vi "InitialiseProbeplan.vi"() -> ()   [LabVIEW 2018]
doc: "General utility to initialise, generate, test and execute probe plans."
uses:
  general_VIs/globals/QC_MeasurementSetup.vi
  ProbePlanParams.vi
  InstrControl/ProbeStationControl/ProbeStationControl.lvclass
panel:
  in  "Use index as X coord":bool=TRUE
  in  "Continue":bool
  in  "New Sensor":bool
  in  "Single Needle":bool=TRUE
  out "Chuck Up/Down check":bool
  in  "Probe Card Channels":i32=1
  in  "Strip No.":u16(ring)
  out "Probeplan:":string="- Click 'New' to load new Probeplan\n- Use controls to check alignment"
  in  "Region":u16(ring)
  in  "Chuck":bool caption="Chuck\nDOWN"
  in  "New Button":bool
  in  "Jump Button":bool
  # "Probeplan"
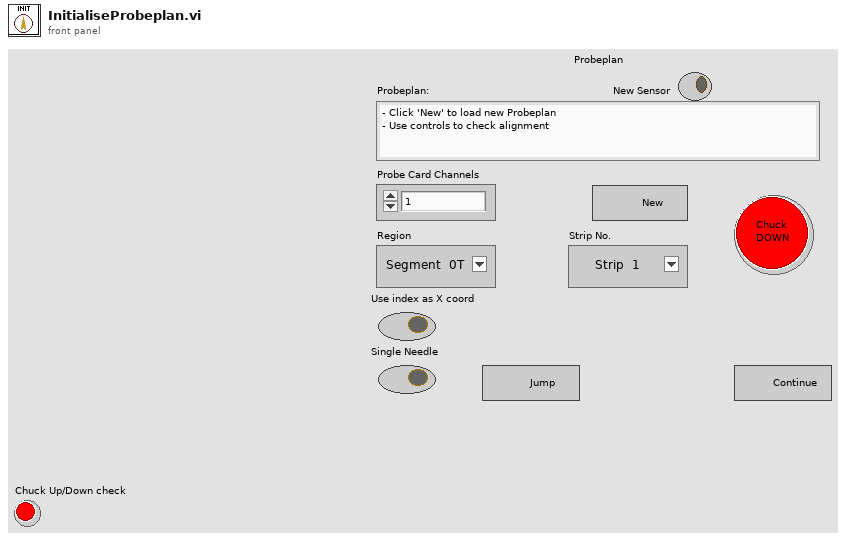
[diagram p1: front panel]
types:
  T1 = cluster{"Bias Supply":refnum<class "SupplyControl.lvclass">, "SMU":refnum<class "SupplyControl.lvclass">, "LCR":refnum<class "LCRControl.lvclass">, "Probe Card Channels":i32, "Bias Voltage [V]":dbl, "First strip":i32, "Last strip":i32, "Base Voltage [V]":dbl, "Base Ramp Step [V]":dbl, "Base Ramp Interval [ms]":u32, "High Voltage [V]":dbl, "High Ramp Step [V]":dbl, "High Ramp Interval [ms]":u32, "Single Needle":bool, "Temperature Readout":enum16{"Read Arduino", "Enter manually"}, "Arduino":refnum<class "ArduinoControl.lvclass">, "Fraction of good strips [%]":dbl, "ProbeStation":refnum<class "ProbeStationControl.lvclass">, "AC frequency [Hz]":i32, "Switching":refnum<class "Switching.lvclass">, "Matrix used?":bool, "Matrix X Channels":cluster{"Bias Supply / SMU LO":i32, "Bias Supply / SMU HI":i32, "CV Box LO":i32, "CV Box HI":i32, "CV Box LO IN":i32, "CV Box HI IN":i32, "Volt meter LO":i32, "Volt meter HI":i32, "Mux1 C1":i32, "Mux1 C2":i32, "Mux2 C1":i32, "Mux2 C2":i32}, "Pinholes Y/N":bool, "Capacitance Y/N":bool, "Resistance Y/N":bool}
  T2 = cluster{"Strip Number OUT":i32, "X0":i32, "Y0":i32, "X1":i32, "Y1":i32, "Xref":dbl, "Yref":dbl, "ProbePlan type":u32, "Inner pads offset":ext, "Outer pads offset":ext, "l_inner":ext, "l_outer":ext, "strip numbering":u16, "Device Orientation":ext, "Stagger offset":i32, "Yoffset":dbl, "Strip pitch":dbl, "Fiducail separation":dbl, "Radius":ext, "Relative strip angles":dbl, "Probeplan description":string, "ProbePlan array":cluster{"Region":string, "ProbePoints":cluster{"X":dbl, "Y":dbl, "Label":string, "CardViable?":bool}[]}[], "Test ProbePoints":cluster{"Regions Enabled":bool[], "From index":u32[], "To index":u32[]}}
  T3 = cluster{"Region":string, "ProbePoints":cluster{"X":dbl, "Y":dbl, "Label":string, "CardViable?":bool}[]}[]
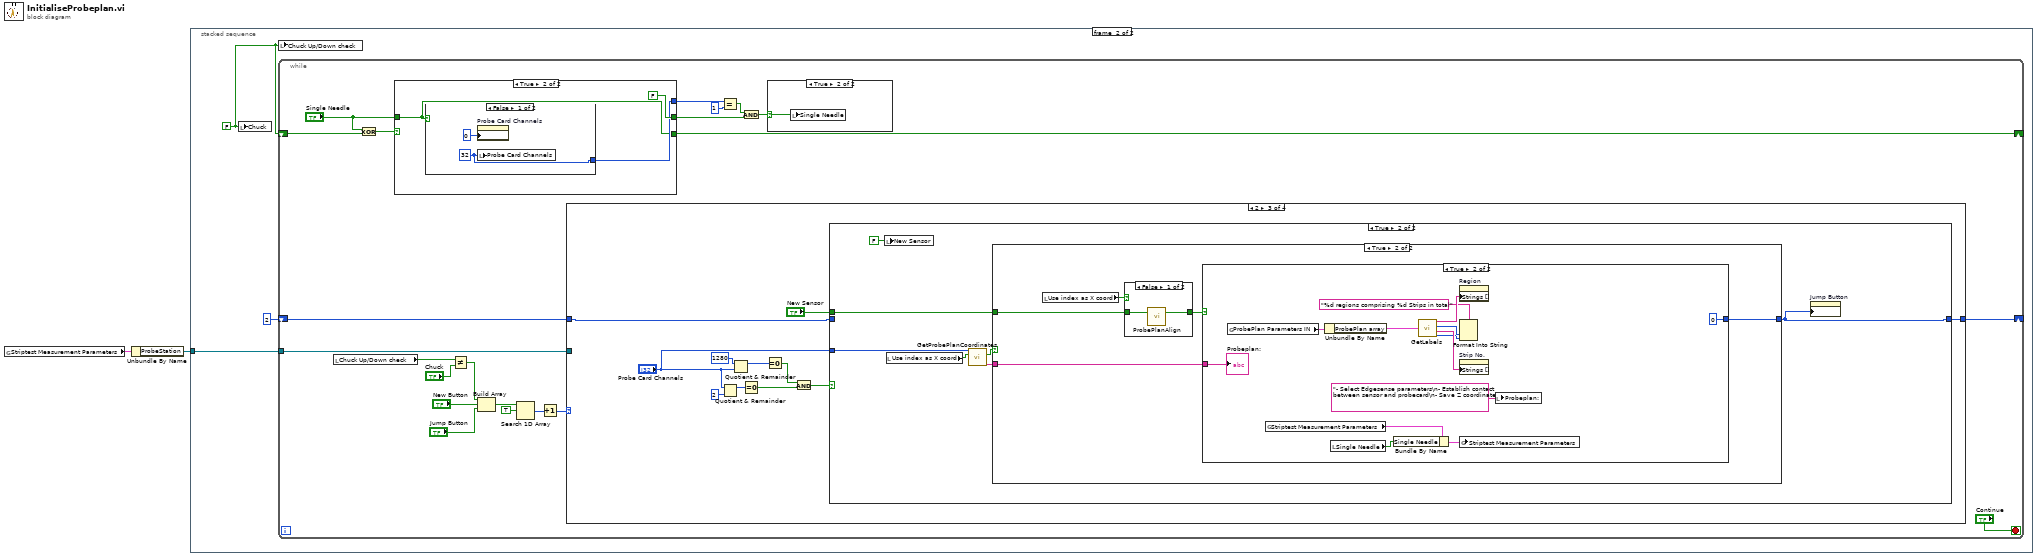
[diagram p0: block diagram]
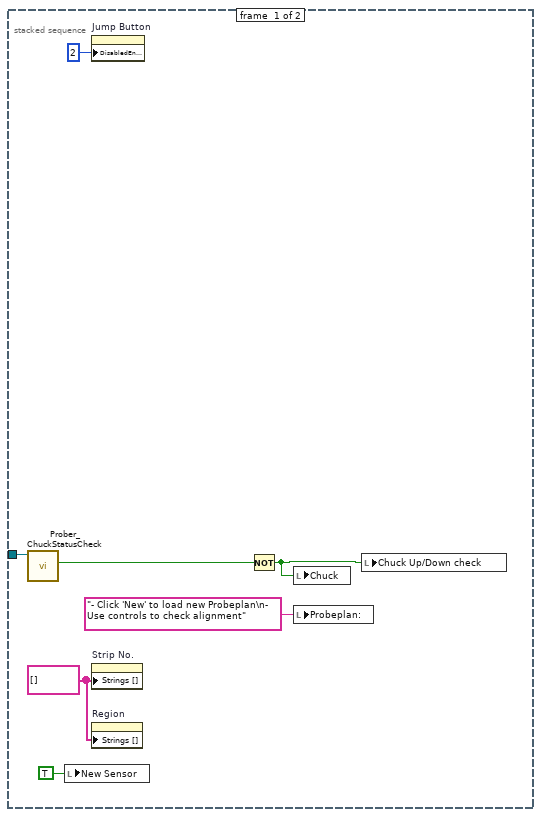
[diagram p2: hidden frame]
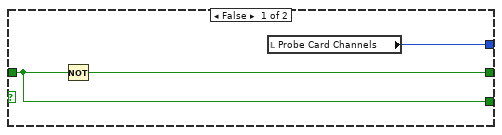
[diagram p4: hidden frame]
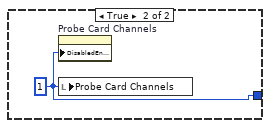
[diagram p5: hidden frame]
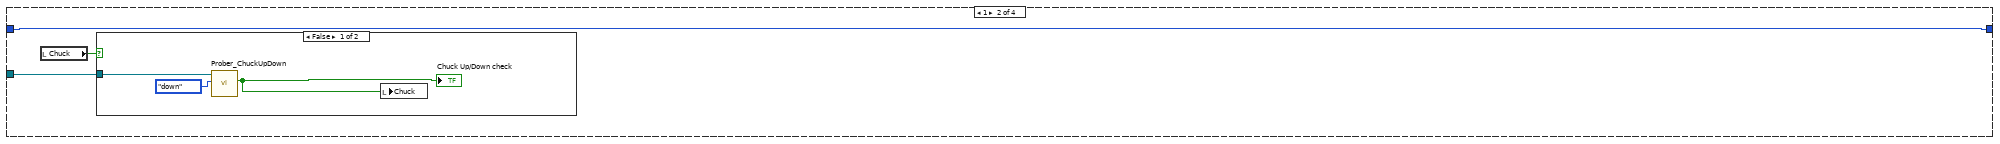
[diagram p7: hidden frame]
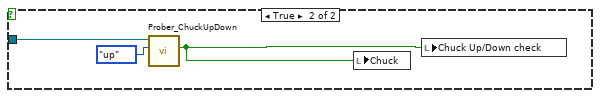
[diagram p8: hidden frame]
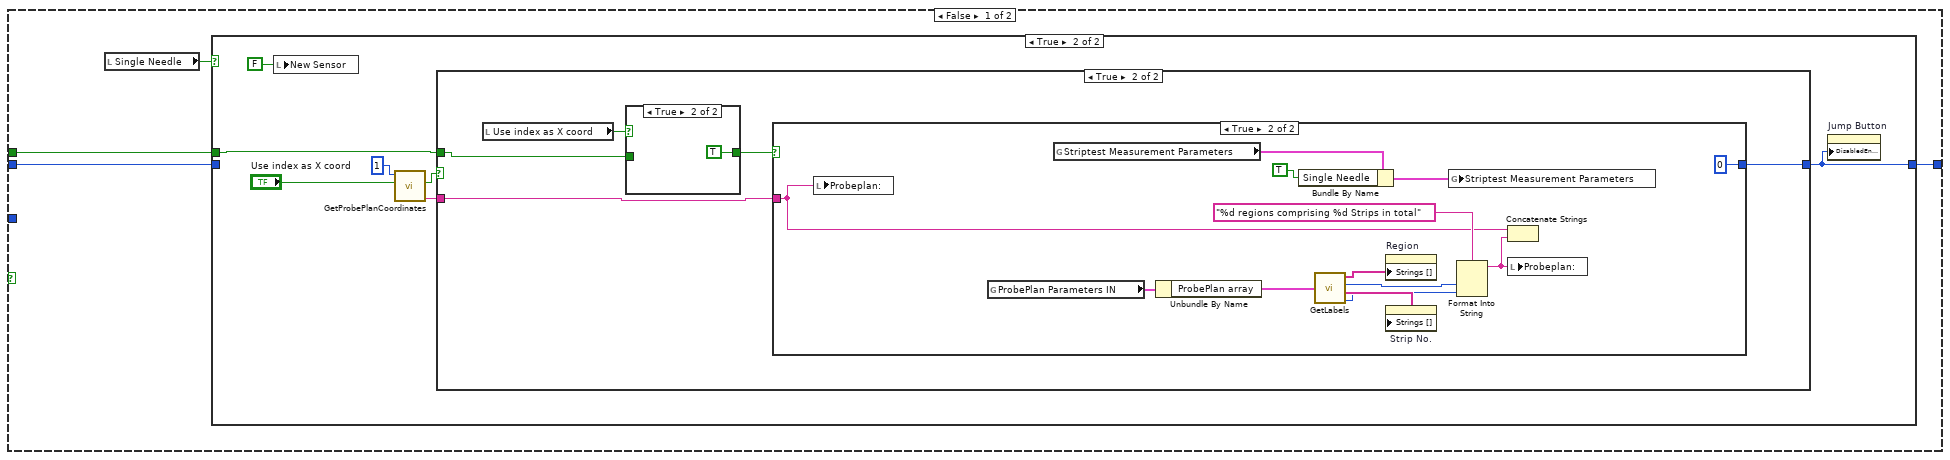
[diagram p9: hidden frame]
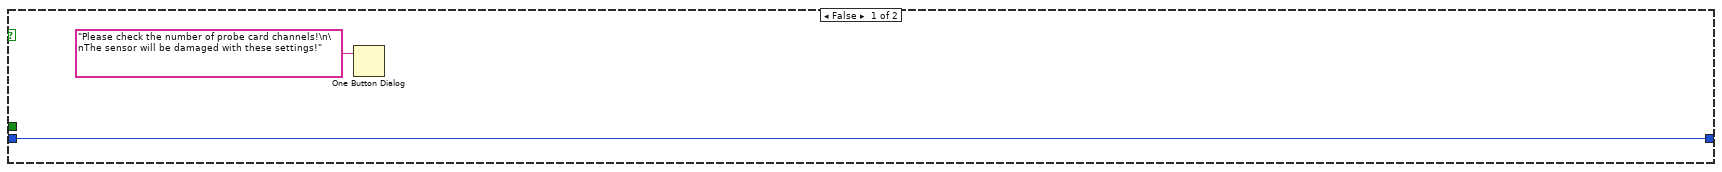
[diagram p10: hidden frame]
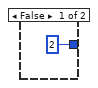
[diagram p11: hidden frame]
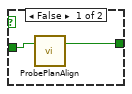
[diagram p12: hidden frame]
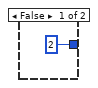
[diagram p13: hidden frame]
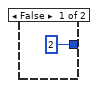
[diagram p14: hidden frame]
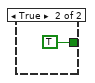
[diagram p15: hidden frame]
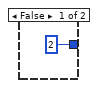
[diagram p16: hidden frame]
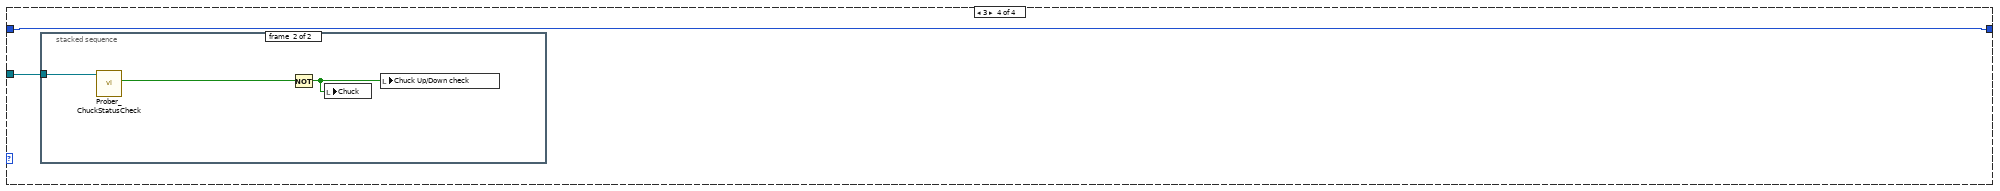
[diagram p17: hidden frame]
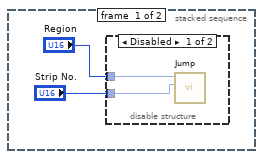
[diagram p18: hidden frame]
diagram:
  n1 = global read "QC_MeasurementSetup.vi" "Striptest Measurement Parameters"() -> (w2:T1)
  n2 = Unbundle By Name(w2) -> ("ProbeStation"=w1:refnum<class "ProbeStationControl.lvclass">)
  n3 = stacked-sequence {
    tunnel: w1 -> [w3 w10]
    frame #0 {
      w7 = string[] []
      n4 = call-dynamic "Prober_ChuckStatusCheck.vi"("ProbeStationControl in"=w3) -> ("Chuck at CONTACT?"=w5:bool)  [unwired: 8 in, 2 out]
      n5 = local write "New Sensor"(TRUE) -> ()
      n6 = property on="Jump Button" class="Bool"("DisabledEnum"=2) -> ()  [unwired: 2 in, 2 out]
      n7 = property on="Strip No." class="Ring (strict)"("Strings []"=w7) -> ()  [unwired: 2 in, 2 out]
      n8 = property on="Region" class="Ring (strict)"("Strings []"=w7) -> ()  [unwired: 2 in, 2 out]
      n9 = Not(x=w5) -> (.not. x?=w4:bool)
      n10 = local write "Chuck"(w4) -> ()
      n11 = local write "Probeplan:"("- Click 'New' to load new Probeplan\n- Use controls to check alignment") -> ()
      n12 = local write "Chuck Up/Down check"(w4) -> ()
    }
    frame #1 {
      w11 = FALSE
      n13 = local write "Chuck"(w11) -> ()
      n14 = local write "Chuck Up/Down check"(w11) -> ()
      n15 = while {
        shift-right: [w27] -> _
        shift-left: 2 -> [w28]
        shift-right: [w15] -> _
        shift-left: w11 -> [w16]
        tunnel: w10 -> [w13]
        stop <- "Continue" stop-if-true
        n16 = local read "Chuck Up/Down check"() -> (w26:bool)
        n17 = Exclusive Or(1:w16, 2:"Single Needle") -> (0:w18:bool)
        n18 = case shown="True" w18 {
          tunnel: [w37 FALSE] -> w21
          tunnel: [w38 w40] -> w19
          tunnel: "Single Needle" -> [w36 w39]
          tunnel: [w36 w39] -> w15
          frame False {
            n19 = Not(x=w36) -> (.not. x?=w37:bool)
            n20 = local read "Probe Card Channels"() -> (w38:i32)
          }
          frame True {
            n21 = case shown="False" w39 {
              tunnel: [w42 w44] -> w40
              frame False {
                w42 = 32
                n22 = property on="Probe Card Channels" class="DigNum (strict)"("DisabledEnum"=0) -> ()  [unwired: 2 in, 2 out]
                n23 = local write "Probe Card Channels"(w42) -> ()
              }
              frame True {
                w44 = 1
                n24 = property on="Probe Card Channels" class="DigNum (strict)"("DisabledEnum"=w44) -> ()  [unwired: 2 in, 2 out]
                n25 = local write "Probe Card Channels"(w44) -> ()
              }
            }
          }
        }
        n26 = Not Equal?(x=w26, y="Chuck") -> (x != y?=w24:bool)
        n27 = Build Array(w24, "New Button", "Jump Button") -> (w33:bool[])
        n28 = Search 1D Array(1D array=w33, element=TRUE) -> (index of element=w34:i32)  [unwired: 1 in]
        n29 = Increment(x=w34) -> (x+1=w29:i32)
        n30 = case shown="2" w29 {
          tunnel: w28 -> [w45 w48 w63 w133]
          tunnel: [w45 w48 w65 w133] -> w27
          tunnel: w13 -> [_ w46 _ w132]
          frame 0, Default {
          }
          frame 1 {
            n31 = local read "Chuck"() -> (w47:bool)
            n32 = case shown="False" w47 {
              tunnel: w46 -> [w50 w52]
              frame False {
                n33 = call-dynamic "Prober_ChuckUpDown.vi"("Direction"=enum16{"up", "down"}."down", "ProbeStationControl in"=w50) -> ("Chuck at CONTACT?"=w51:bool)  [unwired: 7 in, 2 out]
                "Chuck Up/Down check" <- w51
                n34 = local write "Chuck"(w51) -> ()
              }
              frame True {
                n35 = call-dynamic "Prober_ChuckUpDown.vi"("Direction"=enum16{"up", "down"}."up", "ProbeStationControl in"=w52) -> ("Chuck at CONTACT?"=w54:bool)  [unwired: 7 in, 2 out]
                n36 = local write "Chuck"(w54) -> ()
                n37 = local write "Chuck Up/Down check"(w54) -> ()
              }
            }
          }
          frame 2 {
            n38 = Quotient & Remainder(x="Probe Card Channels", y=2) -> (x-y*floor(x/y)=w57:i32)  [unwired: 1 out]
            n39 = Quotient & Remainder(x=1280, y="Probe Card Channels") -> (x-y*floor(x/y)=w64:i32)  [unwired: 1 out]
            n40 = Equal To 0?(x=w57) -> (x = 0?=w56:bool)
            n41 = Equal To 0?(x=w64) -> (x = 0?=w62:bool)
            n42 = And(x=w62, y=w56) -> (x .and. y?=w61:bool)
            n43 = case shown="True" w61 {
              tunnel: "Probe Card Channels" -> [_ w106]
              tunnel: [w68 w105] -> w65
              tunnel: w63 -> [w67 _]
              tunnel: "New Sensor" -> [w66 w104]
              frame False {
                n44 = local read "Single Needle"() -> (w69:bool)
                n45 = case shown="True" w69 {
                  tunnel: [w70 w75] -> w68
                  tunnel: w67 -> [w70 _]
                  tunnel: w66 -> [_ w74]
                  frame False {
                    n46 = One Button Dialog(message="Please check the number of probe card channels!\n\nThe sensor will be damaged with these settings!") -> ()  [unwired: 1 in, 1 out]
                  }
                  frame True {
                    n47 = local write "New Sensor"(FALSE) -> ()
                    n48 = call "GetProbePlanCoordinates.vi"("Use index as X coord"="Use index as X coord", "Probe Card Channels"=1) -> ("file path"=w77:string, "OK?"=w78:bool)  [unwired: 5 in, 1 out]
                    n49 = case shown="True" w78 {
                      tunnel: [2 w84] -> w75
                      tunnel: w77 -> [_ w82]
                      tunnel: w74 -> [_ w81]
                      frame False {
                      }
                      frame True {
                        n50 = local read "Use index as X coord"() -> (w80:bool)
                        n51 = case shown="True" w80 {
                          tunnel: [w86 TRUE ("Accept/Quit")] -> w83
                          tunnel: w81 -> [w85 _]
                          frame False {
                            n52 = call "ProbePlanAlign.vi"("New Sensor"=w85) -> ("Accept/Quit"=w86:bool)  [unwired: 2 in]
                          }
                          frame True {
                          }
                        }
                        n53 = case shown="True" w83 {
                          tunnel: [2 0] -> w84
                          tunnel: w82 -> [_ w90]
                          frame False {
                          }
                          frame True {
                            n54 = local write "Probeplan:"(w90) -> ()
                            n55 = global read "ProbePlanParams.vi" "ProbePlan Parameters IN"() -> (w100:T2)
                            n56 = global read "QC_MeasurementSetup.vi" "Striptest Measurement Parameters"() -> (w92:T1)
                            n57 = Unbundle By Name(w100) -> ("ProbePlan array"=w99:T3)
                            n58 = Bundle By Name(cluster=w92, "Single Needle"=TRUE) -> (w91:T1)
                            n59 = call "GetLabels.vi"("Array"=w99) -> ("Region Labels"=w97:string[], "No. of regions"=w96:i32, "Strip Labels"=w98:string[], "No. of Points"=w95:i32)
                            n60 = property on="Region" class="Ring (strict)"("Strings []"=w97) -> ()  [unwired: 2 in, 2 out]
                            n61 = property on="Strip No." class="Ring (strict)"("Strings []"=w98) -> ()  [unwired: 2 in, 2 out]
                            n62 = global write "QC_MeasurementSetup.vi" "Striptest Measurement Parameters"(w91) -> ()
                            n63 = Format Into String(format string="%d regions comprising %d Strips in total", w96, w95) -> (resulting string=w89:string)  [unwired: 2 in, 1 out]
                            n64 = Concatenate Strings(w90, w89) -> ()  [unwired: 1 out]
                            n65 = local write "Probeplan:"(w89) -> ()
                          }
                        }
                      }
                    }
                    n66 = property on="Jump Button" class="Bool"("DisabledEnum"=w75) -> ()  [unwired: 2 in, 2 out]
                  }
                }
              }
              frame True {
                n67 = local write "New Sensor"(FALSE) -> ()
                n68 = local read "Use index as X coord"() -> (w102:bool)
                n69 = call "GetProbePlanCoordinates.vi"("Use index as X coord"=w102, "Probe Card Channels"=w106) -> ("file path"=w107:string, "OK?"=w108:bool)  [unwired: 5 in, 1 out]
                n70 = case shown="True" w108 {
                  tunnel: [2 w114] -> w105
                  tunnel: w107 -> [_ w112]
                  tunnel: w104 -> [_ w111]
                  frame False {
                  }
                  frame True {
                    n71 = local read "Use index as X coord"() -> (w110:bool)
                    n72 = case shown="False" w110 {
                      tunnel: [w116 TRUE ("Accept/Quit")] -> w113
                      tunnel: w111 -> [w115 _]
                      frame False {
                        n73 = call "ProbePlanAlign.vi"("New Sensor"=w115) -> ("Accept/Quit"=w116:bool)  [unwired: 2 in]
                      }
                      frame True {
                      }
                    }
                    n74 = case shown="True" w113 {
                      tunnel: [2 0] -> w114
                      tunnel: w112 -> [_ w130]
                      frame False {
                      }
                      frame True {
                        n75 = global read "ProbePlanParams.vi" "ProbePlan Parameters IN"() -> (w129:T2)
                        n76 = global read "QC_MeasurementSetup.vi" "Striptest Measurement Parameters"() -> (w121:T1)
                        n77 = Unbundle By Name(w129) -> ("ProbePlan array"=w128:T3)
                        n78 = local read "Single Needle"() -> (w119:bool)
                        n79 = Bundle By Name(cluster=w121, "Single Needle"=w119) -> (w120:T1)
                        n80 = call "GetLabels.vi"("Array"=w128) -> ("Region Labels"=w126:string[], "No. of regions"=w125:i32, "Strip Labels"=w127:string[], "No. of Points"=w124:i32)
                        n81 = property on="Region" class="Ring (strict)"("Strings []"=w126) -> ()  [unwired: 2 in, 2 out]
                        n82 = Format Into String(format string="%d regions comprising %d Strips in total", w125, w124) -> ()  [unwired: 2 in, 2 out]
                        n83 = property on="Strip No." class="Ring (strict)"("Strings []"=w127) -> ()  [unwired: 2 in, 2 out]
                        n84 = global write "QC_MeasurementSetup.vi" "Striptest Measurement Parameters"(w120) -> ()
                        n85 = local write "Probeplan:"("- Select Edgesense parameters\n- Establish contact between sensor and probecard\n- Save Z coordinate") -> ()
                        "Probeplan:" <- w130
                      }
                    }
                  }
                }
                n86 = property on="Jump Button" class="Bool"("DisabledEnum"=w105) -> ()  [unwired: 2 in, 2 out]
              }
            }
          }
          frame 3 {
            n87 = stacked-sequence {
              tunnel: w132 -> [_ w138]
              frame #0 {
                n88 = disable-structure shown="Disabled" {
                  disable-tunnel: "Region" -> [w137 _]
                  disable-tunnel: "Strip No." -> [w136 _]
                  frame Disabled {
                    n89 = call "Jump.vi"("Strip No."=w136, "Region"=w137) -> ()  [unwired: 5 in, 1 out]
                  }
                  frame Enabled {
                  }
                }
              }
              frame #1 {
                n90 = call-dynamic "Prober_ChuckStatusCheck.vi"("ProbeStationControl in"=w138) -> ("Chuck at CONTACT?"=w140:bool)  [unwired: 8 in, 2 out]
                n91 = Not(x=w140) -> (.not. x?=w139:bool)
                n92 = local write "Chuck"(w139) -> ()
                n93 = local write "Chuck Up/Down check"(w139) -> ()
              }
            }
          }
        }
        n94 = Equal?(x=w19, y=1) -> (x = y?=w22:bool)
        n95 = And(x=w22, y=w21) -> (x .and. y?=w20:bool)
        n96 = case shown="True" w20 {
          selector: w20 -> [_ w35]
          frame False {
          }
          frame True {
            n97 = local write "Single Needle"(w35) -> ()
          }
        }
      }
    }
  }
